vi "MB ICPCON Param Write Ip addrs.vi"(8 "error in (no error)":errorcluster, 9 "IP address":T2(array[cluster]), 10 "index (0)":i32, 11 "Param Reference":T1) -> (0 "error out":errorcluster, 3 "Param Reference out":T1)   [LabVIEW 2021, in "ICPCON_Param.lvlib"]
uses:
  ICPCON_Param.lvlib
  ICPCON Param.ctl
  Eth timeouts.ctl
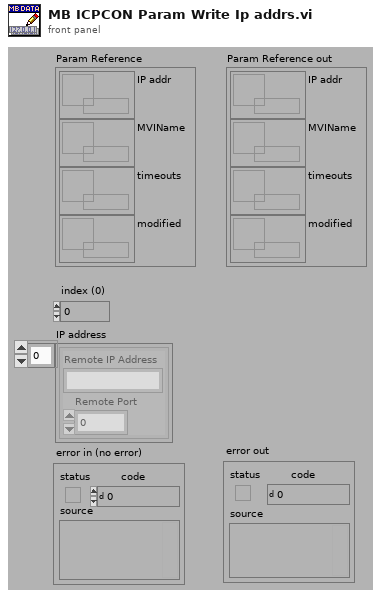
[diagram p1: front panel]
types:
  T1 = typedef "ICPCON_Param.lvlib/ICPCON Param.ctl" = cluster{"IP addr":refnum<data-value>, "MVIName":refnum<data-value>, "timeouts":refnum<data-value>, "modified":refnum<data-value>}
  T2 = cluster{"Remote IP Address":string, "Remote Port":u16}[]
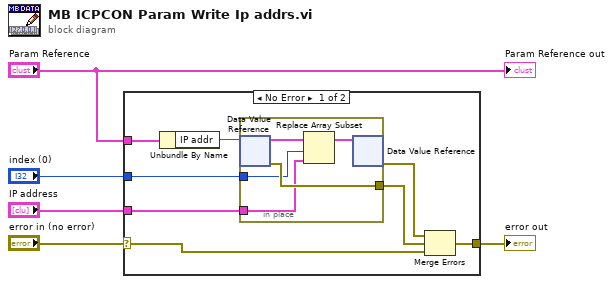
[diagram p0: block diagram]
diagram:
  n1 = case shown="No Error" "error in (no error)" {
    selector: "error in (no error)" -> [w6 w19]
    tunnel: [w11 w19] -> w4
    tunnel: "index (0)" -> [w13 _]
    tunnel: "Param Reference" -> [w12 _]
    tunnel: "IP address" -> [w10 _]
    frame No Error {
      n2 = Unbundle By Name(w12) -> ("IP addr"=w7:refnum<data-value>)
      n3 = in-place {
        in-place-border: w13 -> [w15]
        in-place-border: [w18] -> w8
        in-place-border: w10 -> [w14]
        n4 = in-place-dvr #1(w7) -> (w17:T2, w18:errorcluster)
        n5 = Replace Array Subset(array=w17, new element=w14, index=w15) -> (w16:T2)
        n6 = in-place-dvr #1(w16) -> (w9:errorcluster)  [unwired: 1 out]
      }
      n7 = Merge Errors(w9, w8, w6) -> (w11:errorcluster)
    }
    frame Error {
    }
  }
  "error out" <- w4
  "Param Reference out" <- "Param Reference"
